vi "Build Transfer Group.vi"(8 "error in (no error)":errorcluster, 9 "inline?":bool, 10 "Transfer Group in":refnum<class "Transfer Group.lvclass">, 11 "Buffer Converter in":refnum<class "Buffer Converter.lvclass">) -> (0 "error out":errorcluster, 2 "Transfer Group out":refnum<class "Transfer Group.lvclass">, 3 "Buffer Converter out":refnum<class "Buffer Converter.lvclass">)   [LabVIEW 2017, in "DSF Core.lvlib" / "Buffer Converter.lvclass"]
uses:
  Buffer Converter.lvclass
  Transfer Group/Transfer Group.lvclass
  Transfer Group/Transfer Group.lvclass/Transfer Group.ctl
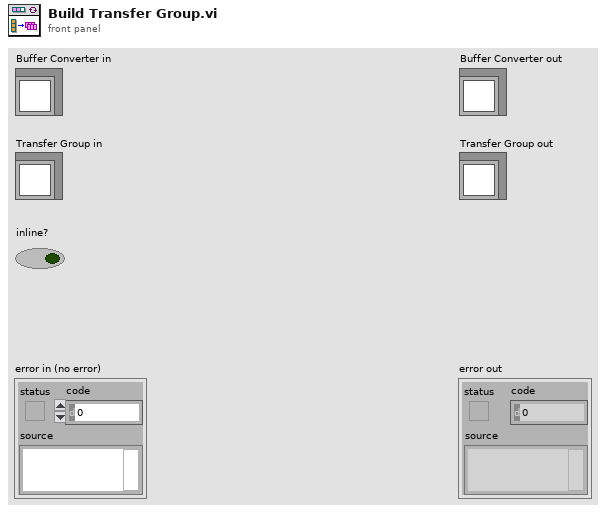
[diagram p1: front panel]
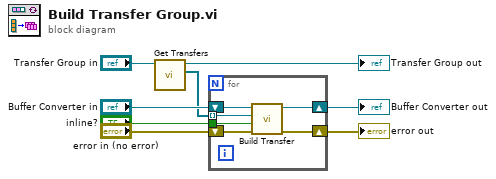
[diagram p0: block diagram]
diagram:
  n1 = call "Get Transfers.vi"("Transfer Group in"="Transfer Group in") -> ("Transfers"=w6:refnum<class "Transfer.lvclass">[], "Transfer Group out"=→"Transfer Group out":refnum<class "Transfer Group.lvclass">)  [unwired: 9 in]
  n2 = for {
    tunnel: w6 -> [w10] mode=indexing
    shift-right: [w11] -> w5
    shift-left: "Buffer Converter in" -> [w12]
    shift-right: [w13] -> w4
    shift-left: "error in (no error)" -> [w14]
    tunnel: "inline?" -> [w9]
    n3 = call "Build Transfer.vi"("error in (no error)"=w14, "inline?"=w9, "Transfer"=w10, "Buffer Converter in"=w12) -> ("error out"=w13:errorcluster, "Buffer Converter out"=w11:refnum<class "Buffer Converter.lvclass">)  [unwired: 6 in]
  }
  "error out" <- w4
  "Buffer Converter out" <- w5
